vi "MSI_Image_overlap.vi"() -> ()   [LabVIEW 2016]
uses:
  <vilib>/vision/NI_Vision_Development_Module.lvlib
panel:
  in  "Angle (degrees)":sgl format="%.2f"
  in  "Transparency":u8 max=80 step=1
  in  "stop":bool
  in  "Open":bool
  in  "Current rotation":sgl format="%.2f"
  out "Overlayed Image":T1(plugin-control)
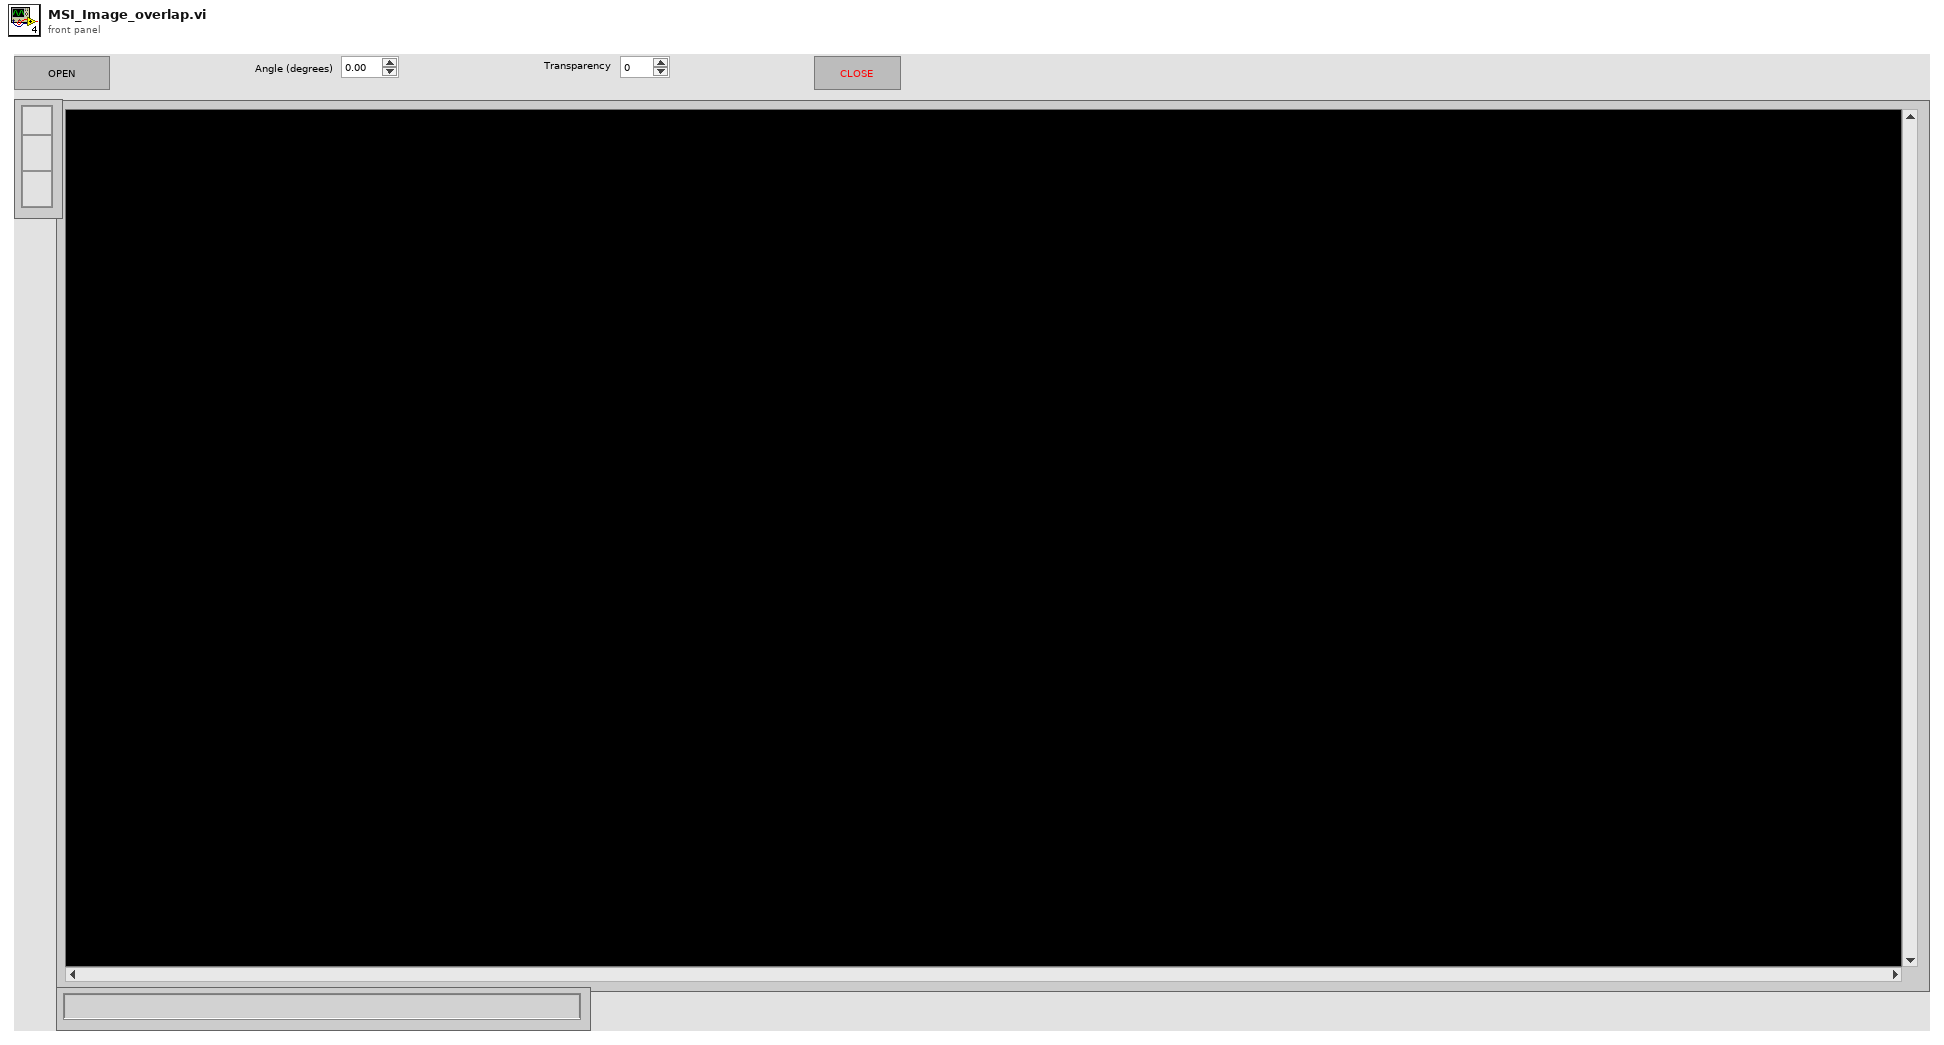
[diagram p1: front panel]
types:
  T1 = typedef "IMAQ Image.ctl" = refnum<image>
  T2 = cluster{"Blue or Luma":u8, "Green or Sat Plane":u8, "Red or Hue Plane":u8, "Alpha":u8}
  T3 = typedef "Image Type" = u32
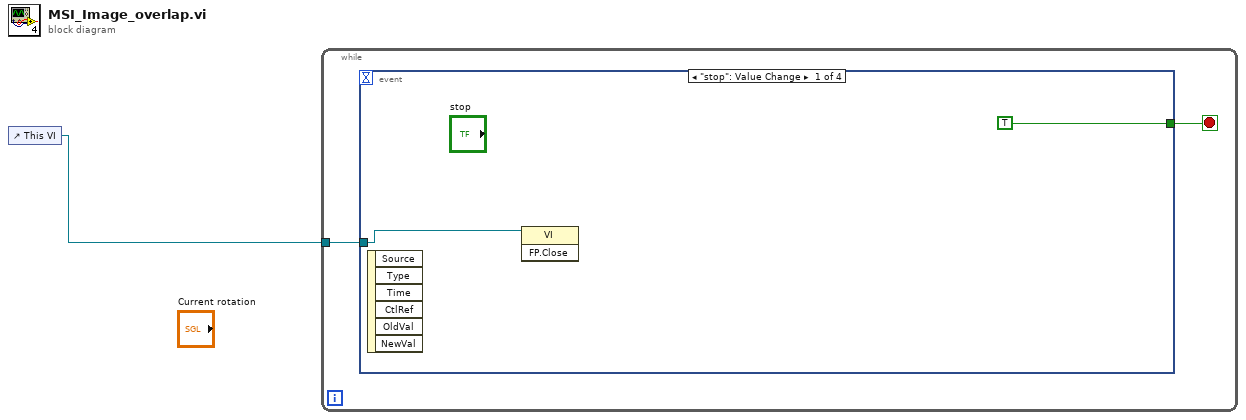
[diagram p0: block diagram]
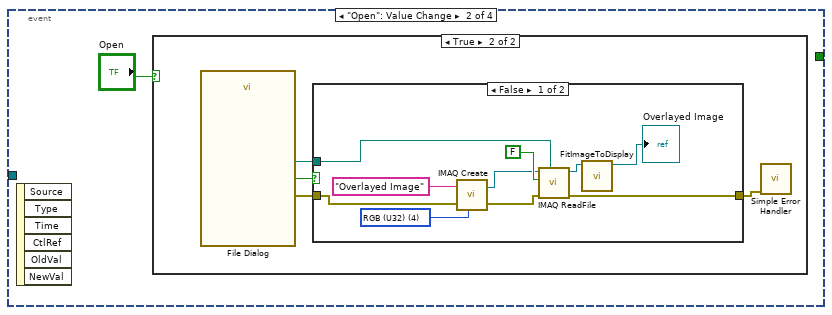
[diagram p2: hidden frame]
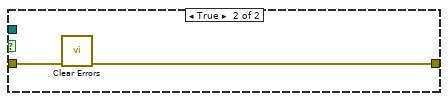
[diagram p4: hidden frame]
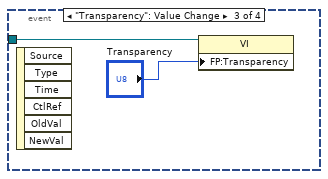
[diagram p5: hidden frame]
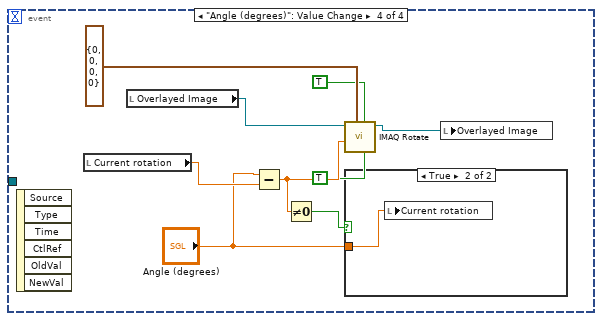
[diagram p6: hidden frame]
diagram:
  n1 = control-ref of="This VI"() -> (w1:refnum<vi>)
  n2 = while {
    tunnel: w1 -> [w2]
    stop <- w3 stop-if-true
    n3 = event shown="[0] \"stop\": Value Change" {
      selector: _ -> [_ _ _ _]
      dyn-events: _ -> [_ _ _ _]
      timeout: _ -> [_ _ _ _]
      tunnel: [TRUE ("stop") _ _ _] -> w3
      tunnel: w2 -> [w4 _ w23 _]
      event "stop": Value Change {
        n4 = event-data() -> ()  [unwired: 1 in, 6 out]
        n5 = invoke class="VI" method="FP.Close"(reference=w4) -> ()  [unwired: 2 in, 3 out]
      }
      event "Open": Value Change {
        n6 = event-data() -> ()  [unwired: 1 in, 6 out]
        n7 = case shown="True" "Open" {
          frame False {
          }
          frame True {
            n8 = call "File Dialog"() -> ("selected path"=w8:path, "cancelled"=w9:bool, "error out"=w10:errorcluster)  [unwired: 12 in, 1 out]
            n9 = case shown="False" w9 {
              tunnel: w8 -> [w20 _]
              tunnel: w10 -> [w11 w22]
              tunnel: [w17 w21] -> w7
              frame False {
                w16 = T3 4 items=["Grayscale (U8)", "Grayscale (I16)", "Grayscale (SGL)", "Complex (CSG)", "RGB (U32)", "HSL (U32)", "RGB (U64)", "Grayscale (U16)"] ("Image Type")
                n10 = call "IMAQ Create"("Image Name"="Overlayed Image", "Image Type"=w16, "error in (no error)"=w11) -> ("New Image"=w14:T1, "error out"=w12:errorcluster)  [unwired: 2 in]
                n11 = call "IMAQ ReadFile"("File Path"=w20, "error in (no error)"=w12, "Load Color Palette? (No)"=FALSE, "Image"=w14) -> ("error out"=w17:errorcluster, "Image Out"=w19:T1)  [unwired: 3 in, 3 out]
                n12 = call "FitImageToDisplay.vi"("Image"=w19) -> ("Image (dup)"=→"Overlayed Image":T1)  [unwired: 9 in]
              }
              frame True {
                n13 = call <vilib>:"Clear Errors.vi"("error in (no error)"=w22) -> ("error out"=w21:errorcluster)  [unwired: 5 in, 1 out]
              }
            }
            n14 = call <vilib>:"Simple Error Handler.vi"("error in (no error)"=w7) -> ()  [unwired: 4 in, 5 out]
          }
        }
      }
      event "Transparency": Value Change {
        n15 = event-data() -> ()  [unwired: 1 in, 6 out]
        n16 = property class="VI"(reference=w23, "FP:Transparency"="Transparency") -> ()  [unwired: 1 in, 2 out]
      }
      event "Angle (degrees)": Value Change {
        n17 = event-data() -> ()  [unwired: 1 in, 6 out]
        n18 = local read "Current rotation"() -> (w29:sgl)
        n19 = local read "Overlayed Image"() -> (w33:T1)
        n20 = Subtract(x="Angle (degrees)", y=w29) -> (x-y=w27:sgl)
        n21 = Not Equal To 0?(x=w27) -> (x != 0?=w26:bool)
        n22 = call "IMAQ Rotate"("Use Bilinear Interpolation"=TRUE, "Maintain Size"=TRUE, "Color Replace Value"=T2 {"Blue or Luma"=0, "Green or Sat Plane"=0, "Red or Hue Plane"=0, "Alpha"=0}, "Angle (degrees)"=w27, "Image Src"=w33) -> ("Image Dst Out"=w32:T1)  [unwired: 5 in, 1 out]
        n23 = case shown="True" w26 {
          tunnel: "Angle (degrees)" -> [_ w34]
          frame False {
          }
          frame True {
            n24 = local write "Current rotation"(w34) -> ()
          }
        }
        n25 = local write "Overlayed Image"(w32) -> ()
      }
    }
  }
